vi "Check User Timestamps FIFO Overflow.vi"(8 "error in (no error)":errorcluster, 11 "FPGA Ref in":refnum<k20>) -> (0 "error out":errorcluster, 2 "User Timestamp FIFO Overflow":bool, 3 "FPGA Ref out":refnum<k20>)   [LabVIEW 2025]
uses:
  <vilib>/Utility/error.llb/Error Cluster From Error Code.vi
  <vilib>/rvi/errors/niLvFpgaAdjustHostInterfaceError.vi
  <vilib>/rvi/interface/nirviReadWriteControl/nirviReadWriteControl.xnode
  NiFpgaLv.dll
  <vilib>/rvi/interface/Simulation/niFpgaSimulationCallBeginRW.vi
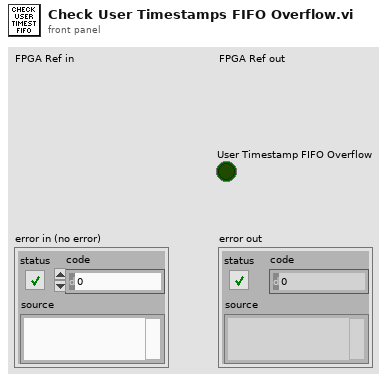
[diagram p1: front panel]
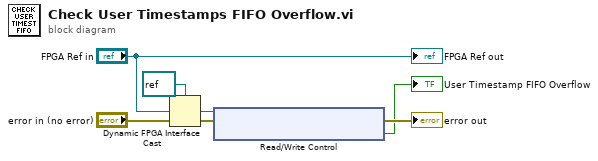
[diagram p0: block diagram]
diagram:
  n1 = Dynamic FPGA Interface Cast(Session In=refnum<k20> refnum ("FPGA VI Reference Out"), Type="FPGA Ref in") -> (Session Out=w2:refnum<k20>)
  n2 = xnode "Read/Write Control"("FPGA VI Reference In"=w2, "error in"="error in (no error)") -> ("error out"=→"error out":errorcluster, "user timestamp fifo overflow"=→"User Timestamp FIFO Overflow":bool)  [unwired: 1 out]
  "FPGA Ref out" <- "FPGA Ref in"
